vi "Query Multi Eval Meas ACLR Limit Check Results.vi"(8 "error in (no error)":errorcluster, 9 "Result Type (Current)":i32(ring) items=["Current", "Average"], 10 "Instance (1)":T2=1, 11 "VISA resource name":refnum<visa-resource-name>) -> (0 "error out":errorcluster, 1 "ACLR Limit Check Results":T1, 2 "Reliability":i32, 3 "VISA resource name out":refnum<visa-resource-name>)   [LabVIEW 2020, in "Rohde&Schwarz CMWXP NR FR1 Measurement.lvlib"]
doc: "Returns the limit check ACLR values for NR standalone, as displayed in the table below the ACLR diagram. The current and average values can be retrieved.\n\nAttributes:\nRSCMWXPNRFR1M_ATTR_QUERY_MULTI_EVAL_MEAS_ACLR_CURRENT_LIMIT_CHECK_RESULTS\nRSCMWXPNRFR1M_ATTR_QUERY_MULTI_EVAL_MEAS_ACLR_AVERAGE_LIMIT_CHECK_RESULTS\n\nRemote-control commands:\nCALCulate:NRSub:MEAS<i>:MEValuation:ACLR:CURRent?\nCALCulate:NRSub:MEAS<i>:MEValuation:ACLR:AVERage?"
uses:
  <instrlib>/Rohde&Schwarz CMWXP NR FR1 Measurement/Rohde&Schwarz CMWXP NR FR1 Measurement.lvlib
  <instrlib>/Rohde&Schwarz CMWXP NR FR1 Measurement/Private/_Instance.ctl
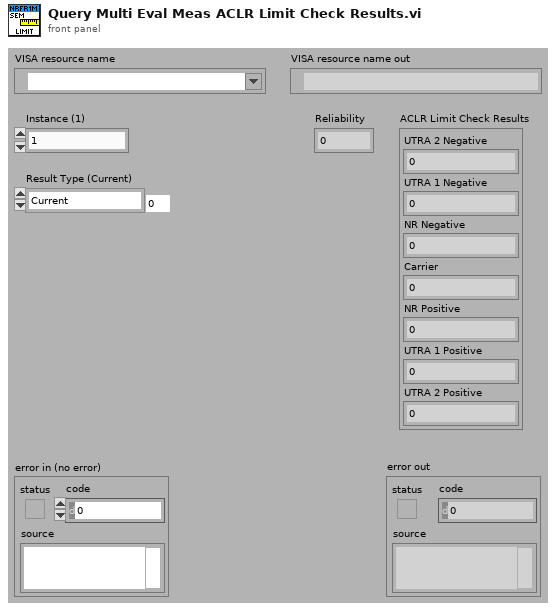
[diagram p1: front panel]
types:
  T1 = cluster{"UTRA 2 Negative":i32, "UTRA 1 Negative":i32, "NR Negative":i32, "Carrier":i32, "NR Positive":i32, "UTRA 1 Positive":i32, "UTRA 2 Positive":i32}
  T2 = typedef "Rohde&Schwarz CMWXP NR FR1 Measurement.lvlib/_Instance.ctl" = i32
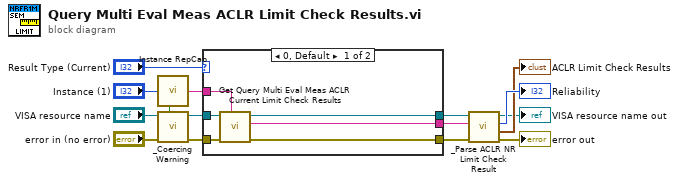
[diagram p0: block diagram]
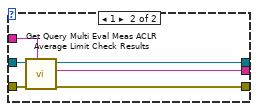
[diagram p2: hidden frame]
diagram:
  n1 = call <instrlib>:"Instance RepCap.vi"("Instance In"="Instance (1)") -> ("In Range?"=w12:bool, "RepCap Identifier Out"=w8:string)  [unwired: 1 in]
  n2 = call <instrlib>:"_Coercing Warning.vi"("In Range?"=w12, "error in (no error)"="error in (no error)", "VISA resource name"="VISA resource name") -> ("error out"=w10:errorcluster, "VISA resource name out"=w11:refnum<visa-resource-name>)  [unwired: 7 in]
  n3 = case shown="0, Default" "Result Type (Current)" {
    tunnel: w11 -> [w21 w27]
    tunnel: w10 -> [w20 w26]
    tunnel: w8 -> [w19 w25]
    tunnel: [w18 w24] -> w7
    tunnel: [w17 w23] -> w6
    tunnel: [w16 w22] -> w5
    frame 0, Default {
      n4 = call "Get Query Multi Eval Meas ACLR Current Limit Check Results"("Repeated Capabilities"=w19, "error in (no error)"=w20, "instrument handle"=w21) -> ("error out"=w18:errorcluster, "Query Multi Eval Meas ACLR Current Limit Check Results"=w17:string, "instrument handle out"=w16:refnum<visa-resource-name>)  [unwired: 6 in]
    }
    frame 1 {
      n5 = call "Get Query Multi Eval Meas ACLR Average Limit Check Results"("Repeated Capabilities"=w25, "error in (no error)"=w26, "instrument handle"=w27) -> ("error out"=w24:errorcluster, "Query Multi Eval Meas ACLR Average Limit Check Results"=w23:string, "instrument handle out"=w22:refnum<visa-resource-name>)  [unwired: 6 in]
    }
  }
  n6 = call <instrlib>:"_Parse ACLR NR Limit Check Result.vi"("error in (no error)"=w7, "Input String"=w6, "VISA resource name"=w5) -> ("error out"=→"error out":errorcluster, "ACLR Limit Check Results"=→"ACLR Limit Check Results":T1, "Reliability"=→"Reliability":i32, "VISA resource name out"=→"VISA resource name out":refnum<visa-resource-name>)  [unwired: 5 in]
